vi "PMBus Block Read.vi"(0 "DevType":i32, 1 "CommandCode":u8, 2 "pByteCount":string, 5 "DevIndex":i32, 7 "PMBusIndex":i32, 9 "SlaveAddr":u8, 11 "error in (no error)":errorcluster, 12 "pData":string, 13 "PEC":u8) -> (4 "pByteCount out":string, 6 "function return":i32, 14 "pData out":string, 15 "error out":errorcluster)   [LabVIEW 2012, in "ControlPMBus.lvlib"]
doc: "int WINAPI PMBus_BlockRead(int DevType,int DevIndex,int PMBusIndex,unsigned char SlaveAddr,unsigned char CommandCode,unsigned char *pData,unsigned char *pByteCount,unsigned char PEC);"
uses:
  ControlPMBus.lvlib
  Ginkgo_Driver.dll
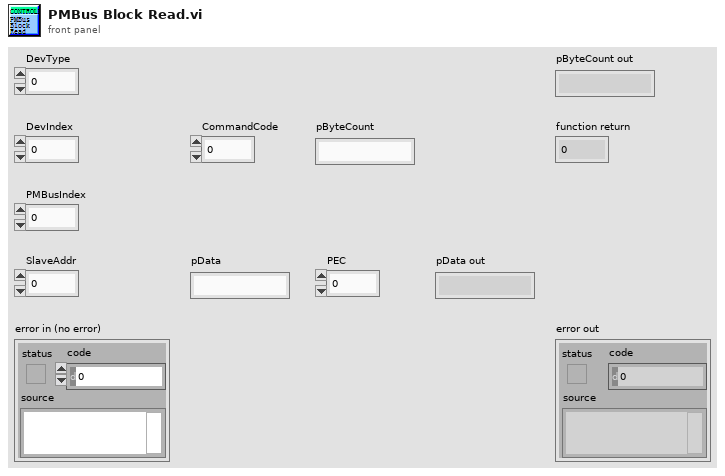
[diagram p1: front panel]
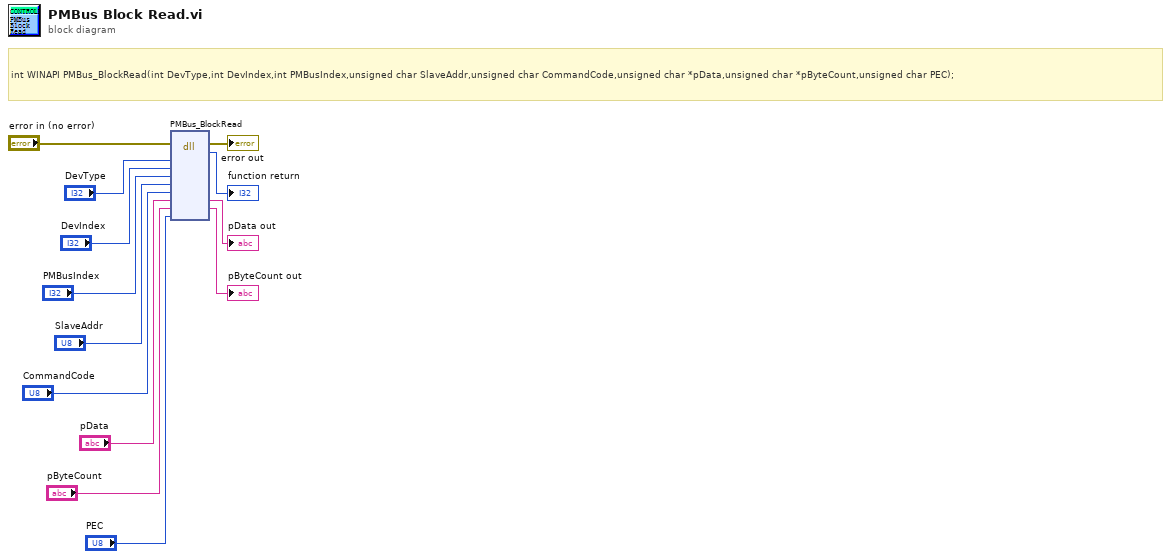
[diagram p0: block diagram]
diagram:
  # "int WINAPI PMBus_BlockRead(int DevType,int DevIndex,int PMBusIndex,unsigned char SlaveAddr,unsigned char CommandCode,unsigned char *pData,unsigned char *pByteCount,unsigned char PEC);"
  n1 = dll-call lib="E:/Project/vt_ginkgo/truck/Ginkgo Driver/vs2010/Ginkgo_USB-I2C_API_v2.0.3.0/lib/labview_64bit/ControlPMBus/Ginkgo_Driver.*" fn="PMBus_BlockRead"(error in="error in (no error)", "DevType"="DevType", "DevIndex"="DevIndex", "PMBusIndex"="PMBusIndex", "SlaveAddr"="SlaveAddr", "CommandCode"="CommandCode", "pData"="pData", "pByteCount"="pByteCount", "PEC"="PEC") -> (error out=→"error out":errorcluster, →"function return":i32, "pData"=→"pData out":string, "pByteCount"=→"pByteCount out":string)  [unwired: 8 in, 1 out]
